vi "Algorithm.vi"() -> ()   [LabVIEW 2016]
uses:
  AdvancedDataStructures/ClassBased/Applications/PriorityQueue/PriorityQueue/PriorityQueue.lvclass
  AdvancedDataStructures/ClassBased/LinkedList/LinkedList.lvclass
  AdvancedDataStructures/ClassBased/Applications/PriorityQueue/PriorityQueue.lvlib
  C:/Users/Rebeca/Documents/Rebeca/Roboime/SSLView/Path Planning/AdvancedDataStructures/ClassBased/Common/BasicSortedList/BasicSortedList/BasicSortedList.lvclass
  C:/Users/Rebeca/Documents/Rebeca/Roboime/SSLView/Path Planning/AdvancedDataStructures/ClassBased/LinkedList/LinkedList.lvclass
  elementGrid.ctl
panel:
  out "Path":dbl[][](array[numeric])
  in  "Nó start 2":dbl[](array[numeric])
  in  "Nó goal 4":dbl[](array[numeric])
  out "element":T1
  in  "GridParameter  3":dbl
  in  "Nó goal 3":dbl[](array[numeric])
  in  "Nó goal 2":dbl[](array[numeric])
  in  "GridParameter  2":dbl
  in  "dy":dbl[](array[numeric])=[1.0, -1.0, 0.0, 0.0, 1.0, -1.0, 1.0, -1.0]
  in  "dx":dbl[](array[numeric])=[0.0, 0.0, 1.0, -1.0, 1.0, 1.0, -1.0, -1.0]
  out "size":i32
  in  "Nó goal":dbl[](array[numeric])
  in  "Nó start":dbl[](array[numeric])
  in  "GridParameter":dbl
  in  "Ystart":dbl format="%#_13g"
  in  "Ygoal":dbl format="%#_13g"
  in  "Xgoal":dbl format="%#_13g"
  in  "Xstart":dbl format="%#_13g"
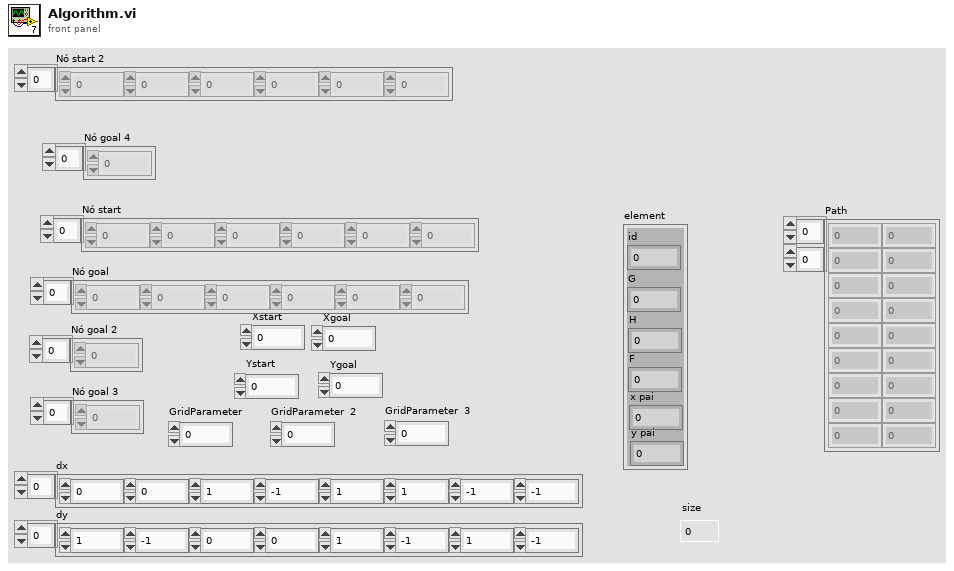
[diagram p1: front panel]
types:
  T1 = typedef "elementGrid.ctl" = cluster{"id":dbl, "G":dbl, "H":dbl, "F":dbl, "x pai":dbl, "y pai":dbl}
  T2 = typedef "grid.ctl" = T1[][]
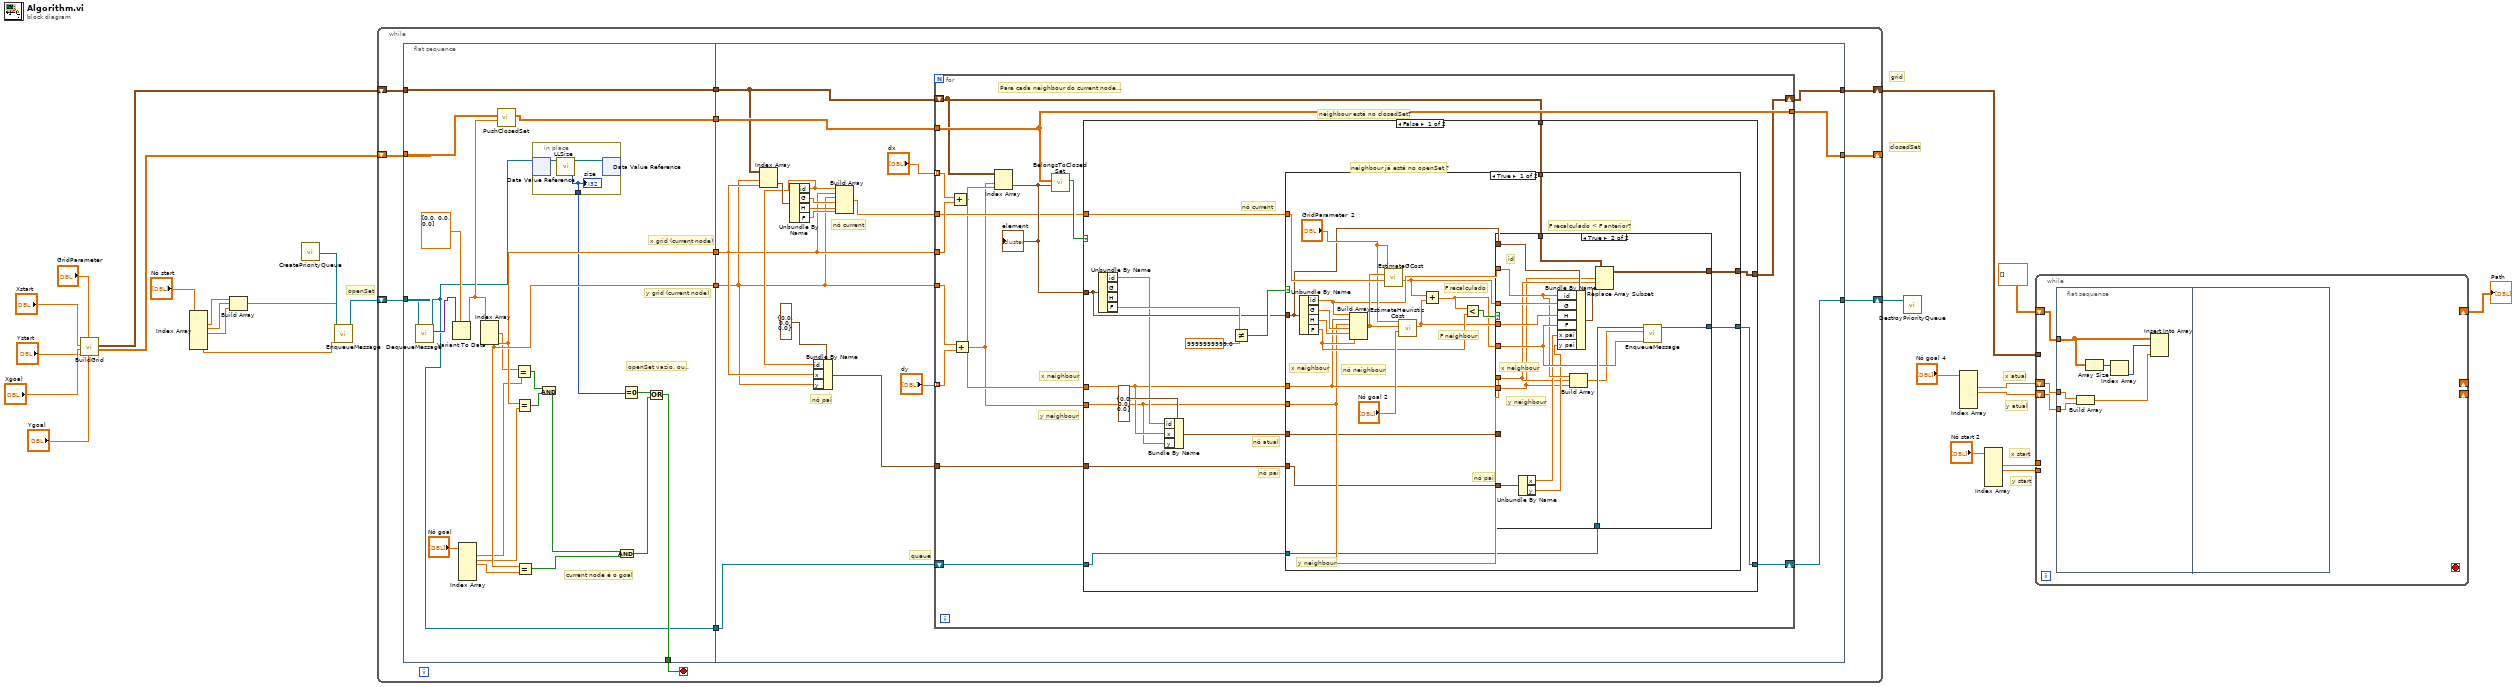
[diagram p0: block diagram]
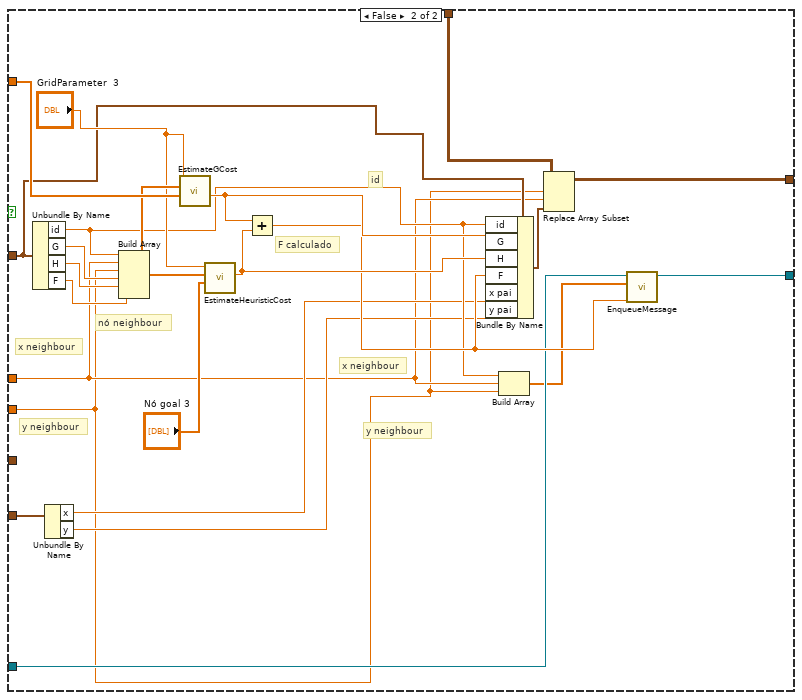
[diagram p3: hidden frame]
diagram:
  # "y atual"
  # "x atual"
  # "y start"
  # "x start"
  # "closedSet"
  # "grid"
  # "openSet"
  n1 = call "BuildGrid.vi"("Ygoal"="Ygoal", "GridParameter"="GridParameter", "Ystart"="Ystart", "Xgoal"="Xgoal", "Xstart"="Xstart") -> ("ClosedSet out"=w13:dbl[][], "grid out"=w14:T2)  [unwired: 3 in, 2 out]
  n2 = Index Array(array="Nó start") -> (element #1=w12:dbl, element #2=w11:dbl, element #3=w18:dbl, element #6=w16:dbl)  [unwired: 6 in, 2 out]
  n3 = Build Array(w12, w11, w18) -> (w17:dbl[])
  n4 = call "CreatePriorityQueue.vi"() -> ("PriorityQueue"=w19:refnum<data-value>)  [unwired: 10 in, 1 out]
  n5 = call "EnqueueMessage.vi"("Priority"=w16, "message"=w17, "queue in"=w19) -> ("queue out"=w15:refnum<data-value>)  [unwired: 7 in, 1 out]
  n6 = while {
    shift-right: [w27] -> w10
    shift-left: w15 -> [w37]
    shift-right: [w26] -> w8
    shift-left: w14 -> [w30]
    shift-right: [w29] -> _
    shift-left: w13 -> [w36]
    stop <- w35 stop-if-true
    n7 = flat-sequence {
      tunnel: w37 -> [w60]
      tunnel: w36 -> [w57]
      tunnel: [w44] -> w35
      tunnel: [w59] -> w34
      tunnel: [w58] -> w33
      tunnel: [w40] -> w32
      tunnel: [w39] -> w31
      tunnel: w30 -> [w39]
      tunnel: [w38] -> w28
      tunnel: w34 -> [w64]
      tunnel: w33 -> [w65]
      tunnel: w32 -> [w79]
      tunnel: w31 -> [w75]
      tunnel: [w78] -> w29
      tunnel: w28 -> [w77]
      tunnel: [w76] -> w27
      tunnel: [w69] -> w26
      frame #0 {
        # "y grid (current node)"
        # "x grid (current node)"
        # "current node é o goal"
        # "openSet vazio, ou.."
        n8 = call "DequeueMessage.vi"("queue in"=w60) -> ("message"=w43:variant, "queue out"=w38:refnum<data-value>)  [unwired: 7 in, 2 out]
        n9 = Variant To Data(type=dbl[] [0.0, 0.0, 0.0] ("New Node"), Variant=w43) -> (data=w45:dbl[])  [unwired: 1 in, 1 out]
        n10 = Index Array(array="Nó goal") -> (element #1=w54:dbl, element #2=w53:dbl, element #3=w52:dbl)  [unwired: 6 in, 3 out]
        n11 = Index Array(array=w45) -> (element #1=w46:dbl, element #2=w58:dbl, element #3=w59:dbl)  [unwired: 3 in]
        n12 = call "PushClosedSet.vi"("Novo nó"=w45, "ClosedSet"=w57) -> ("NewClosedSet"=w40:dbl[][])  [unwired: 9 in]
        n13 = Equal?(x=w46, y=w54) -> (x = y?=w51:bool)
        n14 = Equal?(x=w58, y=w53) -> (x = y?=w50:bool)
        n15 = Equal?(x=w59, y=w52) -> (x = y?=w48:bool)
        n16 = in-place {
          in-place-border: [w61] -> w42
          n17 = in-place-dvr #1(w38) -> (w63:refnum<class "PriorityQueue.lvclass">)  [unwired: 1 out]
          n18 = call "LLSize.vi"("LinkedList in"=w63) -> ("size"=w61:i32, "LinkedList out"=w62:refnum<class "PriorityQueue.lvclass">)  [unwired: 8 in, 1 out]
          "size" <- w61
          n19 = in-place-dvr #1(w62) -> ()  [unwired: 2 out]
        }
        n20 = And(x=w51, y=w50) -> (x .and. y?=w49:bool)
        n21 = And(x=w49, y=w48) -> (x .and. y?=w47:bool)
        n22 = Equal To 0?(x=w42) -> (x = 0?=w41:bool)
        n23 = Or(x=w41, y=w47) -> (x .or. y?=w44:bool)
      }
      frame #1 {
        # "nó pai"
        # "nó current"
        # "queue"
        n24 = Index Array(array=w75, index (row)=w64, index (col)=w65) -> (element=w74:T1)
        n25 = Unbundle By Name(w74) -> ("id"=w67:dbl, "G"=w73:dbl, "H"=w72:dbl, "F"=w71:dbl)
        n26 = Bundle By Name(cluster=cluster{"id":dbl, "x":dbl, "y":dbl} {"id"=0.0, "x"=0.0, "y"=0.0} ("nó atual"), "id"=w67, "x"=w65, "y"=w64) -> (w66:cluster{"id":dbl, "x":dbl, "y":dbl})
        n27 = Build Array(w67, w65, w64, w73, w72, w71) -> (w70:dbl[])
        n28 = for {
          tunnel: "dx" -> [w96] mode=indexing
          tunnel: "dy" -> [w93] mode=indexing
          tunnel: w65 -> [w95]
          tunnel: w64 -> [w94]
          shift-right: [w85] -> w69
          shift-left: w75 -> [w86]
          tunnel: w79 -> [w91]
          tunnel: [w91] -> w78
          shift-right: [w88] -> w76
          shift-left: w77 -> [w90]
          tunnel: w70 -> [w87]
          tunnel: w66 -> [w84]
          # "y neighbour"
          # "x neighbour"
          # "neighbour está no closedSet?"
          # "Para cada neighbour do current node..."
          n29 = Add(x=w96, y=w95) -> (x+y=w83:dbl)
          n30 = Add(x=w94, y=w93) -> (x+y=w82:dbl)
          n31 = Index Array(array=w86, index (row)=w82, index (col)=w83) -> (element=w89:T1)
          "element" <- w89
          n32 = call "BelongsToClosedSet.vi"("neighbour"=w89, "ClosedSet in"=w91) -> ("belongs_to_closedSet"=w92:bool)  [unwired: 9 in]
          n33 = case shown="False" w92 {
            tunnel: w90 -> [w105 w175]
            tunnel: [w104 w175] -> w88
            tunnel: w89 -> [w103 _]
            tunnel: w83 -> [w99 _]
            tunnel: w82 -> [w98 _]
            tunnel: w87 -> [w108 _]
            tunnel: w86 -> [w107 w174]
            tunnel: [w106 w174] -> w85
            tunnel: w84 -> [w102 _]
            frame False {
              # "nó atual"
              # "nó pai"
              # "nó current"
              # "neighbour já está no openSet ?"
              n34 = Unbundle By Name(w103) -> ("id"=w100:dbl, "F"=w111:dbl)  [unwired: 2 out]
              n35 = Bundle By Name(cluster=cluster{"id":dbl, "x":dbl, "y":dbl} {"id"=0.0, "x"=0.0, "y"=0.0} ("nó atual"), "id"=w100, "x"=w99, "y"=w98) -> (w97:cluster{"id":dbl, "x":dbl, "y":dbl})
              n36 = Not Equal?(x=w111, y=9999999999.0) -> (x != y?=w109:bool)
              n37 = case shown="True" w109 {
                tunnel: w103 -> [w117 w162]
                tunnel: w99 -> [w123 w152]
                tunnel: w98 -> [w122 w151]
                tunnel: w108 -> [w130 w171]
                tunnel: w107 -> [w124 w166]
                tunnel: [w116 w161] -> w106
                tunnel: w105 -> [w115 w160]
                tunnel: [w114 w159] -> w104
                tunnel: w102 -> [w112 w155]
                tunnel: w97 -> [w113 _]
                frame True {
                  # "nó pai"
                  # "F recalculado < F anterior?"
                  # "F neighbour"
                  # "F recalculado"
                  # "nó neighbour"
                  # "y neighbour"
                  # "x neighbour"
                  n38 = Unbundle By Name(w117) -> ("id"=w121:dbl, "G"=w132:dbl, "H"=w131:dbl, "F"=w126:dbl)
                  n39 = Build Array(w121, w123, w122, w132, w131, w126) -> (w129:dbl[])
                  n40 = call "EstimateGCost.vi"("Nó pai"=w130, "Nó atual"=w129, "GridParameter"="GridParameter  2") -> ("G_Cost"=w120:dbl)  [unwired: 8 in]
                  n41 = call "EstimateHeuristicCost.vi"("Goal"="Nó goal 2", "Nó atual"=w129, "GridParameter"="GridParameter  2") -> ("Heuristic"=w119:dbl)  [unwired: 8 in]
                  n42 = Add(x=w120, y=w119) -> (x+y=w118:dbl)
                  n43 = Less?(x=w118, y=w126) -> (x < y?=w125:bool)
                  n44 = case shown="True" w125 {
                    tunnel: w124 -> [w133 w150]
                    tunnel: w123 -> [_ w136]
                    tunnel: w122 -> [_ w135]
                    tunnel: w121 -> [_ w142]
                    tunnel: w120 -> [_ w149]
                    tunnel: w119 -> [_ w148]
                    tunnel: w118 -> [_ w143]
                    tunnel: w117 -> [_ w147]
                    tunnel: [w133 w145] -> w116
                    tunnel: w115 -> [w134 w144]
                    tunnel: [w134 w140] -> w114
                    tunnel: w113 -> [_ _]
                    tunnel: w112 -> [_ w139]
                    frame False {
                    }
                    frame True {
                      # "id"
                      # "y neighbour"
                      # "x neighbour"
                      n45 = Unbundle By Name(w139) -> ("x"=w138:dbl, "y"=w137:dbl)
                      n46 = Bundle By Name(cluster=w147, "id"=w142, "G"=w149, "H"=w148, "F"=w143, "x pai"=w138, "y pai"=w137) -> (w146:T1)
                      n47 = Build Array(w142, w136, w135) -> (w141:dbl[])
                      n48 = Replace Array Subset(array=w150, new element=w146, index (row)=w135, index (col)=w136) -> (w145:T2)
                      n49 = call "EnqueueMessage.vi"("Priority"=w143, "message"=w141, "queue in"=w144) -> ("queue out"=w140:refnum<data-value>)  [unwired: 7 in, 1 out]
                    }
                  }
                }
                frame False {
                  # "F calculado"
                  # "id"
                  # "y neighbour"
                  # "x neighbour"
                  # "nó neighbour"
                  # "y neighbour"
                  # "x neighbour"
                  n50 = Unbundle By Name(w162) -> ("id"=w156:dbl, "G"=w173:dbl, "H"=w172:dbl, "F"=w167:dbl)
                  n51 = Unbundle By Name(w155) -> ("x"=w154:dbl, "y"=w153:dbl)
                  n52 = Build Array(w156, w152, w151, w173, w172, w167) -> (w170:dbl[])
                  n53 = call "EstimateGCost.vi"("Nó pai"=w171, "Nó atual"=w170, "GridParameter"="GridParameter  3") -> ("G_Cost"=w165:dbl)  [unwired: 8 in]
                  n54 = call "EstimateHeuristicCost.vi"("Goal"="Nó goal 3", "Nó atual"=w170, "GridParameter"="GridParameter  3") -> ("Heuristic"=w164:dbl)  [unwired: 8 in]
                  n55 = Add(x=w165, y=w164) -> (x+y=w163:dbl)
                  n56 = Bundle By Name(cluster=w162, "id"=w156, "G"=w165, "H"=w164, "F"=w163, "x pai"=w154, "y pai"=w153) -> (w158:T1)
                  n57 = Build Array(w156, w152, w151) -> (w157:dbl[])
                  n58 = Replace Array Subset(array=w166, new element=w158, index (row)=w151, index (col)=w152) -> (w161:T2)
                  n59 = call "EnqueueMessage.vi"("Priority"=w163, "message"=w157, "queue in"=w160) -> ("queue out"=w159:refnum<data-value>)  [unwired: 7 in, 1 out]
                }
              }
            }
            frame True {
            }
          }
        }
      }
    }
  }
  n60 = call "DestroyPriorityQueue.vi"("Queue"=w10) -> ()  [unwired: 10 in, 1 out]
  n61 = Index Array(array="Nó goal 4") -> (element #2=w4:dbl, element #3=w3:dbl)  [unwired: 6 in, 4 out]
  n62 = Index Array(array="Nó start 2") -> (element #2=w6:dbl, element #3=w5:dbl)  [unwired: 6 in, 4 out]
  n63 = while {
    tunnel: w8 -> [_]
    tunnel: w6 -> [_]
    tunnel: w5 -> [_]
    shift-right: _ -> [_]
    shift-left: w4 -> [w177]
    shift-right: _ -> [_]
    shift-left: w3 -> [w176]
    shift-right: [_] -> w1
    shift-left: dbl[][] [] ("Path 2") -> [w178]
    stop <- _ stop-if-true
    n64 = flat-sequence {
      tunnel: w178 -> [w184]
      tunnel: w177 -> [w181]
      tunnel: w176 -> [w180]
      frame #0 {
        n65 = Build Array(w181, w180) -> (w179:dbl[])
        n66 = Array Size(array=w184) -> (size(s)=w183:i32[])
        n67 = Index Array(array=w183) -> (element=w182:i32)  [unwired: 1 in]
        n68 = Insert Into Array(array=w184, index (row)=w182, new element=w179) -> ()  [unwired: 1 in, 1 out]
      }
      frame #1 {
      }
    }
  }
  "Path" <- w1
